vi "Rendering - Font Definition.vi"(11 "Size":i32(ring) items=["Normal", "Small", "Big", "Super Big"]) -> (1 "Exponent Font":T1, 2 "Variable Font":T1, 3 "Number Font":T1, 4 "Matrix Number":T1, 6 "matrix desired font(Application)":T2(ring), 7 "desired font(Application)":T2(ring))   [LabVIEW 2023]
doc: "Define fonts for rendering."
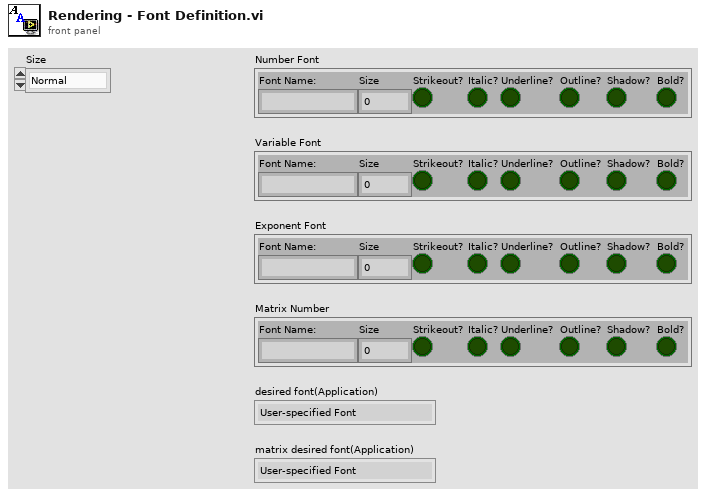
[diagram p1: front panel]
types:
  T1 = cluster{"Font Name:":string, "Size":i16, "Strikeout?":bool, "Italic?":bool, "Underline?":bool, "Outline?":bool, "Shadow?":bool, "Bold?":bool}
  T2 = enum16{"User-specified Font", "Application Font", "System Font", "Dialog Font"}
  T3 = cluster{"Font Name:":string, "Size":i16, "Strikeout?":bool, "Italic?":bool, "Underline?":bool, "Outline?":bool, "Shadow?":bool, "Bold?":bool}[]
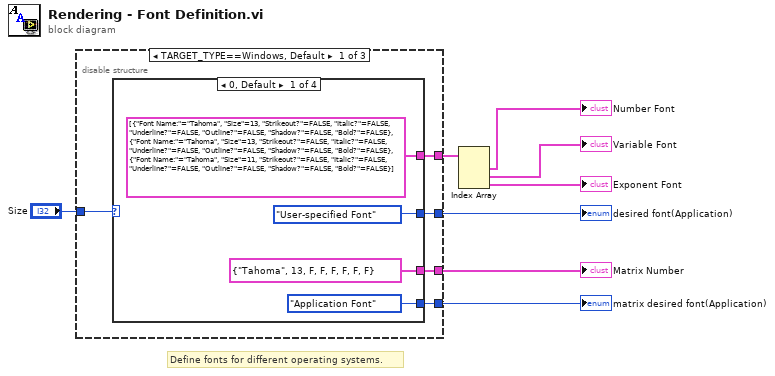
[diagram p0: block diagram]
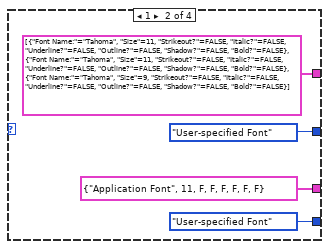
[diagram p2: hidden frame]
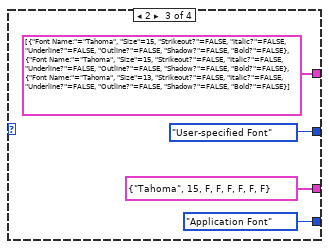
[diagram p3: hidden frame]
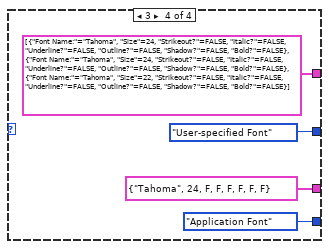
[diagram p4: hidden frame]
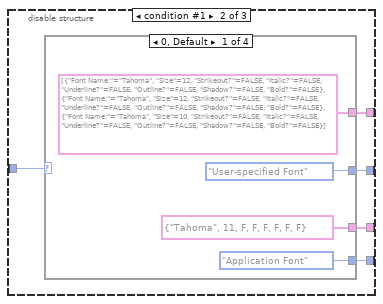
[diagram p5: hidden frame]
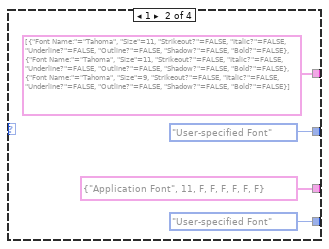
[diagram p6: hidden frame]
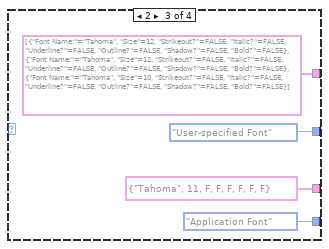
[diagram p7: hidden frame]
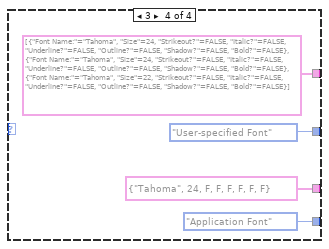
[diagram p8: hidden frame]
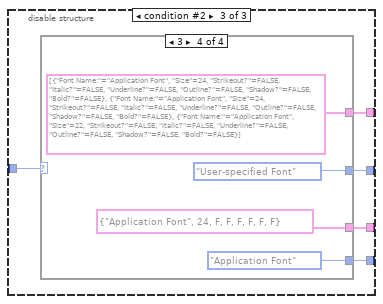
[diagram p9: hidden frame]
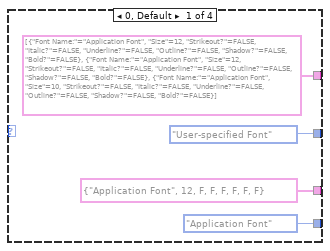
[diagram p10: hidden frame]
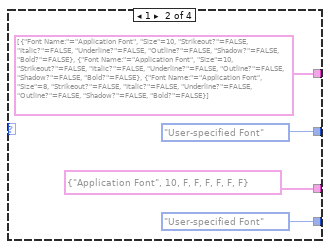
[diagram p11: hidden frame]
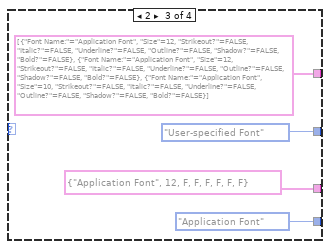
[diagram p12: hidden frame]
diagram:
  # "Define fonts for different operating systems."
  n1 = disable-structure shown="TARGET_TYPE==Windows, Default" {
    disable-tunnel: [w13 w34 w53] -> w1
    disable-tunnel: [w12 w33 w54] -> w5
    disable-tunnel: [w11 w32 w51] -> w4
    disable-tunnel: [w10 w31 w52] -> w3
    disable-tunnel: "Size" -> [w9 w30 w55]
    frame condition #0 (active) {
      n2 = case shown="0, Default" w9 {
        tunnel: [T3 [{"Font Name:"="Tahoma", "Size"=13, "Strikeout?"=FALSE, "Italic?"=FALSE, "Underline?"=FALSE, "Outline?"=FALSE, "Shadow?"=FALSE, "Bold?"=FALSE}, {"Font Name:"="Tahoma", "Size"=13, "Strikeout?"=FALSE, "Italic?"=FALSE, "Underline?"=FALSE, "Outline?"=FALSE, "Shadow?"=FALSE, "Bold?"=FALSE}, {"Font Name:"="Tahoma", "Size"=11, "Strikeout?"=FALSE, "Italic?"=FALSE, "Underline?"=FALSE, "Outline?"=FALSE, "Shadow?"=FALSE, "Bold?"=FALSE}] T3 [{"Font Name:"="Tahoma", "Size"=11, "Strikeout?"=FALSE, "Italic?"=FALSE, "Underline?"=FALSE, "Outline?"=FALSE, "Shadow?"=FALSE, "Bold?"=FALSE}, {"Font Name:"="Tahoma", "Size"=11, "Strikeout?"=FALSE, "Italic?"=FALSE, "Underline?"=FALSE, "Outline?"=FALSE, "Shadow?"=FALSE, "Bold?"=FALSE}, {"Font Name:"="Tahoma", "Size"=9, "Strikeout?"=FALSE, "Italic?"=FALSE, "Underline?"=FALSE, "Outline?"=FALSE, "Shadow?"=FALSE, "Bold?"=FALSE}] T3 [{"Font Name:"="Tahoma", "Size"=15, "Strikeout?"=FALSE, "Italic?"=FALSE, "Underline?"=FALSE, "Outline?"=FALSE, "Shadow?"=FALSE, "Bold?"=FALSE}, {"Font Name:"="Tahoma", "Size"=15, "Strikeout?"=FALSE, "Italic?"=FALSE, "Underline?"=FALSE, "Outline?"=FALSE, "Shadow?"=FALSE, "Bold?"=FALSE}, {"Font Name:"="Tahoma", "Size"=13, "Strikeout?"=FALSE, "Italic?"=FALSE, "Underline?"=FALSE, "Outline?"=FALSE, "Shadow?"=FALSE, "Bold?"=FALSE}] T3 [{"Font Name:"="Tahoma", "Size"=24, "Strikeout?"=FALSE, "Italic?"=FALSE, "Underline?"=FALSE, "Outline?"=FALSE, "Shadow?"=FALSE, "Bold?"=FALSE}, {"Font Name:"="Tahoma", "Size"=24, "Strikeout?"=FALSE, "Italic?"=FALSE, "Underline?"=FALSE, "Outline?"=FALSE, "Shadow?"=FALSE, "Bold?"=FALSE}, {"Font Name:"="Tahoma", "Size"=22, "Strikeout?"=FALSE, "Italic?"=FALSE, "Underline?"=FALSE, "Outline?"=FALSE, "Shadow?"=FALSE, "Bold?"=FALSE}]] -> w13
        tunnel: [T2."User-specified Font" ("desired font(Application)") T2."User-specified Font" ("desired font(Application)") T2."User-specified Font" ("desired font(Application)") T2."User-specified Font" ("desired font(Application)")] -> w12
        tunnel: [T2."Application Font" ("desired font(Application)") T2."User-specified Font" ("desired font(Application)") T2."Application Font" ("desired font(Application)") T2."Application Font" ("desired font(Application)")] -> w11
        tunnel: [T1 {"Font Name:"="Tahoma", "Size"=13, "Strikeout?"=FALSE, "Italic?"=FALSE, "Underline?"=FALSE, "Outline?"=FALSE, "Shadow?"=FALSE, "Bold?"=FALSE} ("Matrix Number") T1 {"Font Name:"="Application Font", "Size"=11, "Strikeout?"=FALSE, "Italic?"=FALSE, "Underline?"=FALSE, "Outline?"=FALSE, "Shadow?"=FALSE, "Bold?"=FALSE} ("Matrix Number") T1 {"Font Name:"="Tahoma", "Size"=15, "Strikeout?"=FALSE, "Italic?"=FALSE, "Underline?"=FALSE, "Outline?"=FALSE, "Shadow?"=FALSE, "Bold?"=FALSE} ("Matrix Number") T1 {"Font Name:"="Tahoma", "Size"=24, "Strikeout?"=FALSE, "Italic?"=FALSE, "Underline?"=FALSE, "Outline?"=FALSE, "Shadow?"=FALSE, "Bold?"=FALSE} ("Matrix Number")] -> w10
        frame 0, Default {
        }
        frame 1 {
        }
        frame 2 {
        }
        frame 3 {
        }
      }
    }
    frame condition #1 {
      n3 = case shown="0, Default" w30 {
        tunnel: [T3 [{"Font Name:"="Tahoma", "Size"=12, "Strikeout?"=FALSE, "Italic?"=FALSE, "Underline?"=FALSE, "Outline?"=FALSE, "Shadow?"=FALSE, "Bold?"=FALSE}, {"Font Name:"="Tahoma", "Size"=12, "Strikeout?"=FALSE, "Italic?"=FALSE, "Underline?"=FALSE, "Outline?"=FALSE, "Shadow?"=FALSE, "Bold?"=FALSE}, {"Font Name:"="Tahoma", "Size"=10, "Strikeout?"=FALSE, "Italic?"=FALSE, "Underline?"=FALSE, "Outline?"=FALSE, "Shadow?"=FALSE, "Bold?"=FALSE}] T3 [{"Font Name:"="Tahoma", "Size"=11, "Strikeout?"=FALSE, "Italic?"=FALSE, "Underline?"=FALSE, "Outline?"=FALSE, "Shadow?"=FALSE, "Bold?"=FALSE}, {"Font Name:"="Tahoma", "Size"=11, "Strikeout?"=FALSE, "Italic?"=FALSE, "Underline?"=FALSE, "Outline?"=FALSE, "Shadow?"=FALSE, "Bold?"=FALSE}, {"Font Name:"="Tahoma", "Size"=9, "Strikeout?"=FALSE, "Italic?"=FALSE, "Underline?"=FALSE, "Outline?"=FALSE, "Shadow?"=FALSE, "Bold?"=FALSE}] T3 [{"Font Name:"="Tahoma", "Size"=12, "Strikeout?"=FALSE, "Italic?"=FALSE, "Underline?"=FALSE, "Outline?"=FALSE, "Shadow?"=FALSE, "Bold?"=FALSE}, {"Font Name:"="Tahoma", "Size"=12, "Strikeout?"=FALSE, "Italic?"=FALSE, "Underline?"=FALSE, "Outline?"=FALSE, "Shadow?"=FALSE, "Bold?"=FALSE}, {"Font Name:"="Tahoma", "Size"=10, "Strikeout?"=FALSE, "Italic?"=FALSE, "Underline?"=FALSE, "Outline?"=FALSE, "Shadow?"=FALSE, "Bold?"=FALSE}] T3 [{"Font Name:"="Tahoma", "Size"=24, "Strikeout?"=FALSE, "Italic?"=FALSE, "Underline?"=FALSE, "Outline?"=FALSE, "Shadow?"=FALSE, "Bold?"=FALSE}, {"Font Name:"="Tahoma", "Size"=24, "Strikeout?"=FALSE, "Italic?"=FALSE, "Underline?"=FALSE, "Outline?"=FALSE, "Shadow?"=FALSE, "Bold?"=FALSE}, {"Font Name:"="Tahoma", "Size"=22, "Strikeout?"=FALSE, "Italic?"=FALSE, "Underline?"=FALSE, "Outline?"=FALSE, "Shadow?"=FALSE, "Bold?"=FALSE}]] -> w34
        tunnel: [T2."User-specified Font" ("desired font(Application)") T2."User-specified Font" ("desired font(Application)") T2."User-specified Font" ("desired font(Application)") T2."User-specified Font" ("desired font(Application)")] -> w33
        tunnel: [T2."Application Font" ("desired font(Application)") T2."User-specified Font" ("desired font(Application)") T2."Application Font" ("desired font(Application)") T2."Application Font" ("desired font(Application)")] -> w32
        tunnel: [T1 {"Font Name:"="Tahoma", "Size"=11, "Strikeout?"=FALSE, "Italic?"=FALSE, "Underline?"=FALSE, "Outline?"=FALSE, "Shadow?"=FALSE, "Bold?"=FALSE} ("Matrix Number") T1 {"Font Name:"="Application Font", "Size"=11, "Strikeout?"=FALSE, "Italic?"=FALSE, "Underline?"=FALSE, "Outline?"=FALSE, "Shadow?"=FALSE, "Bold?"=FALSE} ("Matrix Number") T1 {"Font Name:"="Tahoma", "Size"=11, "Strikeout?"=FALSE, "Italic?"=FALSE, "Underline?"=FALSE, "Outline?"=FALSE, "Shadow?"=FALSE, "Bold?"=FALSE} ("Matrix Number") T1 {"Font Name:"="Tahoma", "Size"=24, "Strikeout?"=FALSE, "Italic?"=FALSE, "Underline?"=FALSE, "Outline?"=FALSE, "Shadow?"=FALSE, "Bold?"=FALSE} ("Matrix Number")] -> w31
        frame 0, Default {
        }
        frame 1 {
        }
        frame 2 {
        }
        frame 3 {
        }
      }
    }
    frame condition #2 {
      n4 = case shown="3" w55 {
        tunnel: [T3 [{"Font Name:"="Application Font", "Size"=12, "Strikeout?"=FALSE, "Italic?"=FALSE, "Underline?"=FALSE, "Outline?"=FALSE, "Shadow?"=FALSE, "Bold?"=FALSE}, {"Font Name:"="Application Font", "Size"=12, "Strikeout?"=FALSE, "Italic?"=FALSE, "Underline?"=FALSE, "Outline?"=FALSE, "Shadow?"=FALSE, "Bold?"=FALSE}, {"Font Name:"="Application Font", "Size"=10, "Strikeout?"=FALSE, "Italic?"=FALSE, "Underline?"=FALSE, "Outline?"=FALSE, "Shadow?"=FALSE, "Bold?"=FALSE}] T3 [{"Font Name:"="Application Font", "Size"=10, "Strikeout?"=FALSE, "Italic?"=FALSE, "Underline?"=FALSE, "Outline?"=FALSE, "Shadow?"=FALSE, "Bold?"=FALSE}, {"Font Name:"="Application Font", "Size"=10, "Strikeout?"=FALSE, "Italic?"=FALSE, "Underline?"=FALSE, "Outline?"=FALSE, "Shadow?"=FALSE, "Bold?"=FALSE}, {"Font Name:"="Application Font", "Size"=8, "Strikeout?"=FALSE, "Italic?"=FALSE, "Underline?"=FALSE, "Outline?"=FALSE, "Shadow?"=FALSE, "Bold?"=FALSE}] T3 [{"Font Name:"="Application Font", "Size"=12, "Strikeout?"=FALSE, "Italic?"=FALSE, "Underline?"=FALSE, "Outline?"=FALSE, "Shadow?"=FALSE, "Bold?"=FALSE}, {"Font Name:"="Application Font", "Size"=12, "Strikeout?"=FALSE, "Italic?"=FALSE, "Underline?"=FALSE, "Outline?"=FALSE, "Shadow?"=FALSE, "Bold?"=FALSE}, {"Font Name:"="Application Font", "Size"=10, "Strikeout?"=FALSE, "Italic?"=FALSE, "Underline?"=FALSE, "Outline?"=FALSE, "Shadow?"=FALSE, "Bold?"=FALSE}] T3 [{"Font Name:"="Application Font", "Size"=24, "Strikeout?"=FALSE, "Italic?"=FALSE, "Underline?"=FALSE, "Outline?"=FALSE, "Shadow?"=FALSE, "Bold?"=FALSE}, {"Font Name:"="Application Font", "Size"=24, "Strikeout?"=FALSE, "Italic?"=FALSE, "Underline?"=FALSE, "Outline?"=FALSE, "Shadow?"=FALSE, "Bold?"=FALSE}, {"Font Name:"="Application Font", "Size"=22, "Strikeout?"=FALSE, "Italic?"=FALSE, "Underline?"=FALSE, "Outline?"=FALSE, "Shadow?"=FALSE, "Bold?"=FALSE}]] -> w53
        tunnel: [T2."User-specified Font" ("desired font(Application)") T2."User-specified Font" ("desired font(Application)") T2."User-specified Font" ("desired font(Application)") T2."User-specified Font" ("desired font(Application)")] -> w54
        tunnel: [T2."Application Font" ("desired font(Application)") T2."User-specified Font" ("desired font(Application)") T2."Application Font" ("desired font(Application)") T2."Application Font" ("desired font(Application)")] -> w51
        tunnel: [T1 {"Font Name:"="Application Font", "Size"=12, "Strikeout?"=FALSE, "Italic?"=FALSE, "Underline?"=FALSE, "Outline?"=FALSE, "Shadow?"=FALSE, "Bold?"=FALSE} ("Matrix Number") T1 {"Font Name:"="Application Font", "Size"=10, "Strikeout?"=FALSE, "Italic?"=FALSE, "Underline?"=FALSE, "Outline?"=FALSE, "Shadow?"=FALSE, "Bold?"=FALSE} ("Matrix Number") T1 {"Font Name:"="Application Font", "Size"=12, "Strikeout?"=FALSE, "Italic?"=FALSE, "Underline?"=FALSE, "Outline?"=FALSE, "Shadow?"=FALSE, "Bold?"=FALSE} ("Matrix Number") T1 {"Font Name:"="Application Font", "Size"=24, "Strikeout?"=FALSE, "Italic?"=FALSE, "Underline?"=FALSE, "Outline?"=FALSE, "Shadow?"=FALSE, "Bold?"=FALSE} ("Matrix Number")] -> w52
        frame 0, Default {
        }
        frame 1 {
        }
        frame 2 {
        }
        frame 3 {
        }
      }
    }
  }
  "desired font(Application)" <- w5
  "matrix desired font(Application)" <- w4
  "Matrix Number" <- w3
  n5 = Index Array(array=w1) -> (element #1=→"Number Font":T1, element #2=→"Variable Font":T1, element #3=→"Exponent Font":T1)  [unwired: 3 in]
